vi "Es.vi"(0 "Reduced Nozzle (A*)":dbl, 1 "Vehicle Volume (Vm)":dbl, 2 "Vehicle Length (Lm)":dbl, 3 "Tunnel Shape Factor (t)":dbl, 4 "Vehicle Frontal Area (Am)":dbl) -> (5 "Induced Velocity due to Jet Expansion (Es)":dbl)   [LabVIEW 2017]
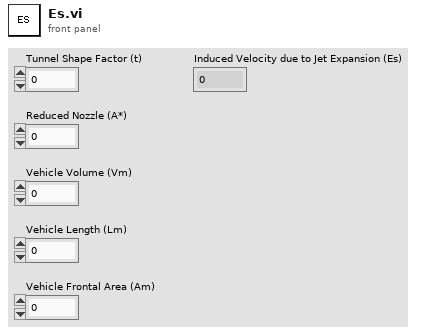
[diagram p1: front panel]
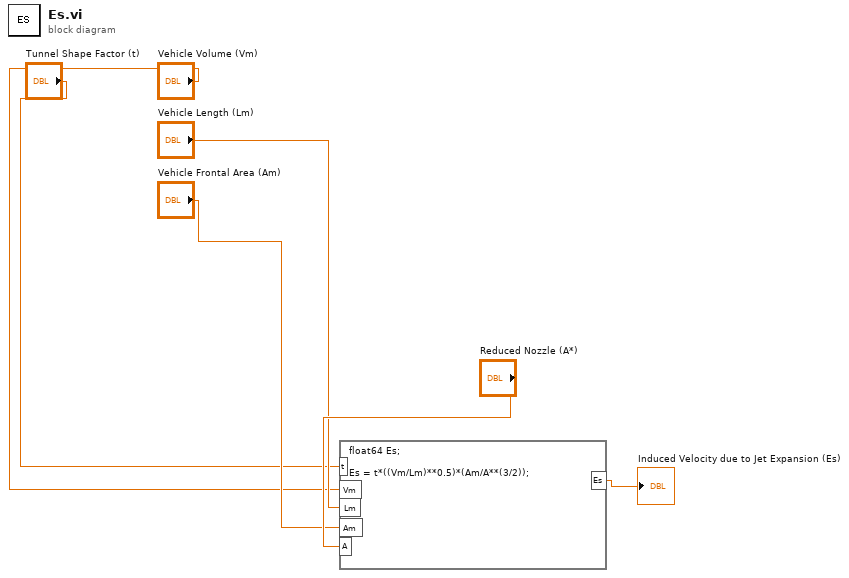
[diagram p0: block diagram]
diagram:
  n1 = formula code="float64 Es;\n\nEs = t*((Vm/Lm)**0.5)*(Am/A**(3/2));"("t"="Tunnel Shape Factor (t)", "Vm"="Vehicle Volume (Vm)", "Lm"="Vehicle Length (Lm)", "Am"="Vehicle Frontal Area (Am)", "A"="Reduced Nozzle (A*)") -> ("Es"=→"Induced Velocity due to Jet Expansion (Es)":dbl)
